vi "Add Item to Tree.vi"(8 "error in (no error)":errorcluster, 9 "Item":T1, 10 "parent tag":string, 11 "TreeControl in":refnum<vi>) -> (0 "error out":errorcluster, 2 "new item tag":string, 3 "TreeControl out":refnum<vi>)   [LabVIEW 2019, in "DSF Configuration Utility.lvlib"]
uses:
  DSF Configuration Utility.lvlib
  Tree Item.ctl
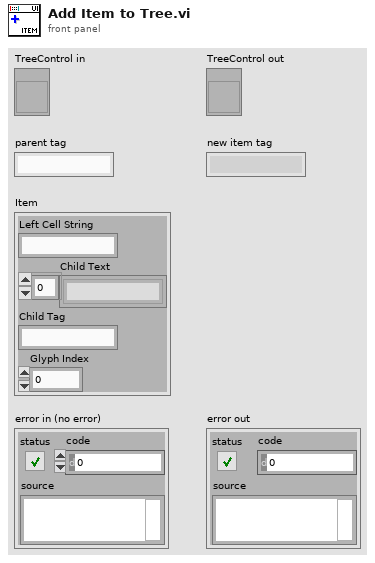
[diagram p1: front panel]
types:
  T1 = typedef "DSF Configuration Utility.lvlib/Tree Item.ctl" = cluster{"Left Cell String":string, "Child Text":string[], "Child Tag":string, "Glyph Index":i32}
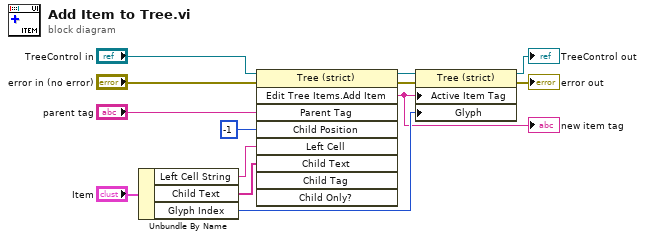
[diagram p0: block diagram]
diagram:
  n1 = Unbundle By Name("Item") -> ("Left Cell String"=w5:string, "Child Text"=w6:string[], "Glyph Index"=w9:i32)
  n2 = invoke class="Tree (strict)" method="Edit Tree Items.Add Item"(reference="TreeControl in", error in="error in (no error)", "Parent Tag"="parent tag", "Child Position"=-1, "Left Cell"=w5, "Child Text"=w6) -> (reference out=w7:refnum<vi>, error out=w12:errorcluster, "Edit Tree Items:Add Item"=w8:string)  [unwired: 3 in, 6 out]
  "new item tag" <- w8
  n3 = property class="Tree (strict)"(reference=w7, error in=w12, "Active Item Tag"=w8, "Glyph"=w9) -> (reference out=→"TreeControl out":refnum<vi>, error out=→"error out":errorcluster)
